vi "Lab Panel V5.28.vi"() -> ()   [LabVIEW 2013] (continued)
                  tunnel: w2122 -> [_ w2132]
                  frame False {
                  }
                  frame True {
                    n1115 = local read "SET LAB01-1"() -> (w2134:T5)
                    n1116 = local read "TDMS LAB01-1"() -> (w2127:refnum<k34>)
                    n1117 = Unbundle(w2134) -> ("CYCLES"=w2125:dbl, "T-RISE mins"=w2131:dbl)  [unwired: 3 out]
                    n1118 = case shown="\"CYCLE TEST\"" w2132 {
                      tunnel: w2131 -> [_ _ w2141]
                      tunnel: [w2136 w2138 w2141] -> w2130
                      tunnel: w2125 -> [w2136 w2138 _]
                      tunnel: ["CHART PASS" "CYCLE PASS" "T-RISE PASS"] -> w2129
                      frame "CHART TEST", Default {
                      }
                      frame "CYCLE TEST" {
                      }
                      frame "T-RISE TEST" {
                      }
                    }
                    n1119 = Unbundle(w2128) -> ("CYCLE"=w2133:dbl)  [unwired: 2 out]
                    n1120 = Increment(x=w2125) -> (x+1=w2126:dbl)
                    n1121 = Greater Or Equal?(x=w2133, y=w2126) -> (x >= y?=w2135:bool)
                    n1122 = case shown="True" w2135 {
                      tunnel: w2130 -> [w2145 _]
                      tunnel: w2129 -> [w2144 _]
                      tunnel: w2128 -> [w2143 _]
                      tunnel: w2127 -> [w2142 _]
                      frame True {
                        n1123 = stacked-sequence {
                          tunnel: w2145 -> [w2149 _]
                          tunnel: w2144 -> [w2147 w2153]
                          tunnel: w2143 -> [_ w2156]
                          tunnel: w2142 -> [w2146 _]
                          frame #0 {
                            n1124 = Build Array(w2147) -> (w2150:string[])
                            n1125 = Build Array(w2149) -> (w2148:dbl[])
                            n1126 = TDMS Write(0:w2146, 5:"TEST PASS", 7:w2150, 9:w2148) -> (15:w2152:errorcluster)  [unwired: 2 in, 3 out]
                            n1127 = local write "data file error"(w2152) -> ()
                          }
                          frame #1 {
                            n1128 = Bundle(cluster=w2156, "STATUS"=w2153) -> (w2154:T4)  [unwired: 2 in]
                            n1129 = local write "RESULT LAB01-1"(TRUE) -> ()
                            n1130 = local write "DISP LAB01-1"(w2154) -> ()
                          }
                        }
                      }
                      frame False {
                      }
                    }
                  }
                }
              }
              frame #1 {
                # "LAB01-2"
                n1131 = Less?(x=w2157, y=2) -> (x < y?=w2160:bool)
                n1132 = local read "DISP LAB01-2"() -> (w2162:T4)
                n1133 = Unbundle(w2162) -> ("STATUS"=w2163:string)  [unwired: 2 out]
                n1134 = Equal?(x=w2163, y="RUN") -> (x = y?=w2159:bool)
                n1135 = And(x=w2159, y=w2160) -> (x .and. y?=w2158:bool)
                n1136 = case shown="True" w2158 {
                  tunnel: w2162 -> [_ w2168]
                  tunnel: w2157 -> [_ w2172]
                  frame False {
                  }
                  frame True {
                    n1137 = local read "SET LAB01-2"() -> (w2174:T5)
                    n1138 = local read "TDMS LAB01-2"() -> (w2167:refnum<k34>)
                    n1139 = Unbundle(w2174) -> ("CYCLES"=w2165:dbl, "T-RISE mins"=w2171:dbl)  [unwired: 3 out]
                    n1140 = case shown="\"T-RISE TEST\"" w2172 {
                      tunnel: w2171 -> [_ _ w2181]
                      tunnel: [w2176 w2178 w2181] -> w2170
                      tunnel: w2165 -> [w2176 w2178 _]
                      tunnel: ["CHART PASS" "CYCLE PASS" "T-RISE PASS"] -> w2169
                      frame "CHART TEST", Default {
                      }
                      frame "CYCLE TEST" {
                      }
                      frame "T-RISE TEST" {
                      }
                    }
                    n1141 = Unbundle(w2168) -> ("CYCLE"=w2173:dbl)  [unwired: 2 out]
                    n1142 = Increment(x=w2165) -> (x+1=w2166:dbl)
                    n1143 = Greater Or Equal?(x=w2173, y=w2166) -> (x >= y?=w2175:bool)
                    n1144 = case shown="True" w2175 {
                      tunnel: w2170 -> [w2185 _]
                      tunnel: w2169 -> [w2184 _]
                      tunnel: w2168 -> [w2183 _]
                      tunnel: w2167 -> [w2182 _]
                      frame True {
                        n1145 = stacked-sequence {
                          tunnel: w2185 -> [w2189 _]
                          tunnel: w2184 -> [w2187 w2193]
                          tunnel: w2183 -> [_ w2196]
                          tunnel: w2182 -> [w2186 _]
                          frame #0 {
                            n1146 = Build Array(w2187) -> (w2190:string[])
                            n1147 = Build Array(w2189) -> (w2188:dbl[])
                            n1148 = TDMS Write(0:w2186, 5:"TEST PASS", 7:w2190, 9:w2188) -> (15:w2192:errorcluster)  [unwired: 2 in, 3 out]
                            n1149 = local write "data file error"(w2192) -> ()
                          }
                          frame #1 {
                            n1150 = Bundle(cluster=w2196, "STATUS"=w2193) -> (w2194:T4)  [unwired: 2 in]
                            n1151 = local write "RESULT LAB01-2"(TRUE) -> ()
                            n1152 = local write "DISP LAB01-2"(w2194) -> ()
                          }
                        }
                      }
                      frame False {
                      }
                    }
                  }
                }
              }
              frame #2 {
                # "LAB02-1"
                n1153 = Less?(x=w2197, y=2) -> (x < y?=w2200:bool)
                n1154 = local read "DISP LAB02-1"() -> (w2202:T4)
                n1155 = Unbundle(w2202) -> ("STATUS"=w2203:string)  [unwired: 2 out]
                n1156 = Equal?(x=w2203, y="RUN") -> (x = y?=w2199:bool)
                n1157 = And(x=w2199, y=w2200) -> (x .and. y?=w2198:bool)
                n1158 = case shown="True" w2198 {
                  tunnel: w2202 -> [_ w2208]
                  tunnel: w2197 -> [_ w2212]
                  frame False {
                  }
                  frame True {
                    n1159 = local read "SET LAB02-1"() -> (w2214:T5)
                    n1160 = local read "TDMS LAB02-1"() -> (w2207:refnum<k34>)
                    n1161 = Unbundle(w2208) -> ("CYCLE"=w2213:dbl)  [unwired: 2 out]
                    n1162 = Unbundle(w2214) -> ("CYCLES"=w2205:dbl, "T-RISE mins"=w2211:dbl)  [unwired: 3 out]
                    n1163 = case shown="\"T-RISE TEST\"" w2212 {
                      tunnel: w2211 -> [_ _ w2221]
                      tunnel: [w2216 w2218 w2221] -> w2210
                      tunnel: w2205 -> [w2216 w2218 _]
                      tunnel: ["CHART PASS" "CYCLE PASS" "T-RISE PASS"] -> w2209
                      frame "CHART TEST", Default {
                      }
                      frame "CYCLE TEST" {
                      }
                      frame "T-RISE TEST" {
                      }
                    }
                    n1164 = Increment(x=w2205) -> (x+1=w2206:dbl)
                    n1165 = Greater Or Equal?(x=w2213, y=w2206) -> (x >= y?=w2215:bool)
                    n1166 = case shown="True" w2215 {
                      tunnel: w2210 -> [w2225 _]
                      tunnel: w2209 -> [w2224 _]
                      tunnel: w2208 -> [w2223 _]
                      tunnel: w2207 -> [w2222 _]
                      frame True {
                        n1167 = stacked-sequence {
                          tunnel: w2225 -> [w2229 _]
                          tunnel: w2224 -> [w2227 w2233]
                          tunnel: w2223 -> [_ w2236]
                          tunnel: w2222 -> [w2226 _]
                          frame #0 {
                            n1168 = Build Array(w2227) -> (w2230:string[])
                            n1169 = Build Array(w2229) -> (w2228:dbl[])
                            n1170 = TDMS Write(0:w2226, 5:"TEST PASS", 7:w2230, 9:w2228) -> (15:w2232:errorcluster)  [unwired: 2 in, 3 out]
                            n1171 = local write "data file error"(w2232) -> ()
                          }
                          frame #1 {
                            n1172 = Bundle(cluster=w2236, "STATUS"=w2233) -> (w2234:T4)  [unwired: 2 in]
                            n1173 = local write "RESULT LAB02-1"(TRUE) -> ()
                            n1174 = local write "DISP LAB02-1"(w2234) -> ()
                          }
                        }
                      }
                      frame False {
                      }
                    }
                  }
                }
              }
              frame #3 {
                # "LAB02-2"
                n1175 = Less?(x=w2237, y=2) -> (x < y?=w2240:bool)
                n1176 = local read "DISP LAB02-2"() -> (w2242:T4)
                n1177 = Unbundle(w2242) -> ("STATUS"=w2243:string)  [unwired: 2 out]
                n1178 = Equal?(x=w2243, y="RUN") -> (x = y?=w2239:bool)
                n1179 = And(x=w2239, y=w2240) -> (x .and. y?=w2238:bool)
                n1180 = case shown="True" w2238 {
                  tunnel: w2242 -> [_ w2248]
                  tunnel: w2237 -> [_ w2252]
                  frame False {
                  }
                  frame True {
                    n1181 = local read "SET LAB02-2"() -> (w2254:T5)
                    n1182 = local read "TDMS LAB02-2"() -> (w2247:refnum<k34>)
                    n1183 = Unbundle(w2248) -> ("CYCLE"=w2253:dbl)  [unwired: 2 out]
                    n1184 = Unbundle(w2254) -> ("CYCLES"=w2245:dbl, "T-RISE mins"=w2251:dbl)  [unwired: 3 out]
                    n1185 = case shown="\"T-RISE TEST\"" w2252 {
                      tunnel: w2251 -> [_ _ w2261]
                      tunnel: [w2256 w2258 w2261] -> w2250
                      tunnel: w2245 -> [w2256 w2258 _]
                      tunnel: ["CHART PASS" "CYCLE PASS" "T-RISE PASS"] -> w2249
                      frame "CHART TEST", Default {
                      }
                      frame "CYCLE TEST" {
                      }
                      frame "T-RISE TEST" {
                      }
                    }
                    n1186 = Increment(x=w2245) -> (x+1=w2246:dbl)
                    n1187 = Greater Or Equal?(x=w2253, y=w2246) -> (x >= y?=w2255:bool)
                    n1188 = case shown="True" w2255 {
                      tunnel: w2250 -> [w2265 _]
                      tunnel: w2249 -> [w2264 _]
                      tunnel: w2248 -> [w2263 _]
                      tunnel: w2247 -> [w2262 _]
                      frame True {
                        n1189 = stacked-sequence {
                          tunnel: w2265 -> [w2269 _]
                          tunnel: w2264 -> [w2267 w2273]
                          tunnel: w2263 -> [_ w2276]
                          tunnel: w2262 -> [w2266 _]
                          frame #0 {
                            n1190 = Build Array(w2267) -> (w2270:string[])
                            n1191 = Build Array(w2269) -> (w2268:dbl[])
                            n1192 = TDMS Write(0:w2266, 5:"TEST PASS", 7:w2270, 9:w2268) -> (15:w2272:errorcluster)  [unwired: 2 in, 3 out]
                            n1193 = local write "data file error"(w2272) -> ()
                          }
                          frame #1 {
                            n1194 = Bundle(cluster=w2276, "STATUS"=w2273) -> (w2274:T4)  [unwired: 2 in]
                            n1195 = local write "RESULT LAB02-2"(TRUE) -> ()
                            n1196 = local write "DISP LAB02-2"(w2274) -> ()
                          }
                        }
                      }
                      frame False {
                      }
                    }
                  }
                }
              }
              frame #4 {
                # "LAB03-1"
                n1197 = Less?(x=w2277, y=2) -> (x < y?=w2280:bool)
                n1198 = local read "DISP LAB03-1"() -> (w2282:T4)
                n1199 = Unbundle(w2282) -> ("STATUS"=w2283:string)  [unwired: 2 out]
                n1200 = Equal?(x=w2283, y="RUN") -> (x = y?=w2279:bool)
                n1201 = And(x=w2279, y=w2280) -> (x .and. y?=w2278:bool)
                n1202 = case shown="True" w2278 {
                  tunnel: w2282 -> [_ w2288]
                  tunnel: w2277 -> [_ w2292]
                  frame False {
                  }
                  frame True {
                    n1203 = local read "SET LAB03-1"() -> (w2294:T5)
                    n1204 = local read "TDMS LAB03-1"() -> (w2287:refnum<k34>)
                    n1205 = Unbundle(w2288) -> ("CYCLE"=w2293:dbl)  [unwired: 2 out]
                    n1206 = Unbundle(w2294) -> ("CYCLES"=w2285:dbl, "T-RISE mins"=w2291:dbl)  [unwired: 3 out]
                    n1207 = case shown="\"T-RISE TEST\"" w2292 {
                      tunnel: w2291 -> [_ _ w2301]
                      tunnel: [w2296 w2298 w2301] -> w2290
                      tunnel: w2285 -> [w2296 w2298 _]
                      tunnel: ["CHART PASS" "CYCLE PASS" "T-RISE PASS"] -> w2289
                      frame "CHART TEST", Default {
                      }
                      frame "CYCLE TEST" {
                      }
                      frame "T-RISE TEST" {
                      }
                    }
                    n1208 = Increment(x=w2285) -> (x+1=w2286:dbl)
                    n1209 = Greater Or Equal?(x=w2293, y=w2286) -> (x >= y?=w2295:bool)
                    n1210 = case shown="True" w2295 {
                      tunnel: w2290 -> [w2305 _]
                      tunnel: w2289 -> [w2304 _]
                      tunnel: w2288 -> [w2303 _]
                      tunnel: w2287 -> [w2302 _]
                      frame True {
                        n1211 = stacked-sequence {
                          tunnel: w2305 -> [w2309 _]
                          tunnel: w2304 -> [w2307 w2313]
                          tunnel: w2303 -> [_ w2316]
                          tunnel: w2302 -> [w2306 _]
                          frame #0 {
                            n1212 = Build Array(w2307) -> (w2310:string[])
                            n1213 = Build Array(w2309) -> (w2308:dbl[])
                            n1214 = TDMS Write(0:w2306, 5:"TEST PASS", 7:w2310, 9:w2308) -> (15:w2312:errorcluster)  [unwired: 2 in, 3 out]
                            n1215 = local write "data file error"(w2312) -> ()
                          }
                          frame #1 {
                            n1216 = Bundle(cluster=w2316, "STATUS"=w2313) -> (w2314:T4)  [unwired: 2 in]
                            n1217 = local write "RESULT LAB03-1"(TRUE) -> ()
                            n1218 = local write "DISP LAB03-1"(w2314) -> ()
                          }
                        }
                      }
                      frame False {
                      }
                    }
                  }
                }
              }
              frame #5 {
                # "LAB03-2"
                n1219 = Less?(x=w2317, y=2) -> (x < y?=w2320:bool)
                n1220 = local read "DISP LAB03-2"() -> (w2322:T4)
                n1221 = Unbundle(w2322) -> ("STATUS"=w2323:string)  [unwired: 2 out]
                n1222 = Equal?(x=w2323, y="RUN") -> (x = y?=w2319:bool)
                n1223 = And(x=w2319, y=w2320) -> (x .and. y?=w2318:bool)
                n1224 = case shown="True" w2318 {
                  tunnel: w2322 -> [_ w2328]
                  tunnel: w2317 -> [_ w2332]
                  frame False {
                  }
                  frame True {
                    n1225 = local read "SET LAB03-2"() -> (w2334:T5)
                    n1226 = local read "TDMS LAB03-2"() -> (w2327:refnum<k34>)
                    n1227 = Unbundle(w2328) -> ("CYCLE"=w2333:dbl)  [unwired: 2 out]
                    n1228 = Unbundle(w2334) -> ("CYCLES"=w2325:dbl, "T-RISE mins"=w2331:dbl)  [unwired: 3 out]
                    n1229 = case shown="\"T-RISE TEST\"" w2332 {
                      tunnel: w2331 -> [_ _ w2341]
                      tunnel: [w2336 w2338 w2341] -> w2330
                      tunnel: w2325 -> [w2336 w2338 _]
                      tunnel: ["CHART PASS" "CYCLE PASS" "T-RISE PASS"] -> w2329
                      frame "CHART TEST", Default {
                      }
                      frame "CYCLE TEST" {
                      }
                      frame "T-RISE TEST" {
                      }
                    }
                    n1230 = Increment(x=w2325) -> (x+1=w2326:dbl)
                    n1231 = Greater Or Equal?(x=w2333, y=w2326) -> (x >= y?=w2335:bool)
                    n1232 = case shown="True" w2335 {
                      tunnel: w2330 -> [w2345 _]
                      tunnel: w2329 -> [w2344 _]
                      tunnel: w2328 -> [w2343 _]
                      tunnel: w2327 -> [w2342 _]
                      frame True {
                        n1233 = stacked-sequence {
                          tunnel: w2345 -> [w2349 _]
                          tunnel: w2344 -> [w2347 w2353]
                          tunnel: w2343 -> [_ w2356]
                          tunnel: w2342 -> [w2346 _]
                          frame #0 {
                            n1234 = Build Array(w2347) -> (w2350:string[])
                            n1235 = Build Array(w2349) -> (w2348:dbl[])
                            n1236 = TDMS Write(0:w2346, 5:"TEST PASS", 7:w2350, 9:w2348) -> (15:w2352:errorcluster)  [unwired: 2 in, 3 out]
                            n1237 = local write "data file error"(w2352) -> ()
                          }
                          frame #1 {
                            n1238 = Bundle(cluster=w2356, "STATUS"=w2353) -> (w2354:T4)  [unwired: 2 in]
                            n1239 = local write "RESULT LAB03-2"(TRUE) -> ()
                            n1240 = local write "DISP LAB03-2"(w2354) -> ()
                          }
                        }
                      }
                      frame False {
                      }
                    }
                  }
                }
              }
              frame #6 {
                # "LAB04-1"
                n1241 = Less?(x=w2357, y=2) -> (x < y?=w2360:bool)
                n1242 = local read "DISP LAB04-1"() -> (w2362:T4)
                n1243 = Unbundle(w2362) -> ("STATUS"=w2363:string)  [unwired: 2 out]
                n1244 = Equal?(x=w2363, y="RUN") -> (x = y?=w2359:bool)
                n1245 = And(x=w2359, y=w2360) -> (x .and. y?=w2358:bool)
                n1246 = case shown="True" w2358 {
                  tunnel: w2362 -> [_ w2368]
                  tunnel: w2357 -> [_ w2372]
                  frame False {
                  }
                  frame True {
                    n1247 = local read "SET LAB04-1"() -> (w2374:T5)
                    n1248 = local read "TDMS LAB04-1"() -> (w2367:refnum<k34>)
                    n1249 = Unbundle(w2368) -> ("CYCLE"=w2373:dbl)  [unwired: 2 out]
                    n1250 = Unbundle(w2374) -> ("CYCLES"=w2365:dbl, "T-RISE mins"=w2371:dbl)  [unwired: 3 out]
                    n1251 = case shown="\"T-RISE TEST\"" w2372 {
                      tunnel: w2371 -> [_ _ w2381]
                      tunnel: [w2376 w2378 w2381] -> w2370
                      tunnel: w2365 -> [w2376 w2378 _]
                      tunnel: ["CHART PASS" "CYCLE PASS" "T-RISE PASS"] -> w2369
                      frame "CHART TEST", Default {
                      }
                      frame "CYCLE TEST" {
                      }
                      frame "T-RISE TEST" {
                      }
                    }
                    n1252 = Increment(x=w2365) -> (x+1=w2366:dbl)
                    n1253 = Greater Or Equal?(x=w2373, y=w2366) -> (x >= y?=w2375:bool)
                    n1254 = case shown="True" w2375 {
                      tunnel: w2370 -> [w2385 _]
                      tunnel: w2369 -> [w2384 _]
                      tunnel: w2368 -> [w2383 _]
                      tunnel: w2367 -> [w2382 _]
                      frame True {
                        n1255 = stacked-sequence {
                          tunnel: w2385 -> [w2389 _]
                          tunnel: w2384 -> [w2387 w2393]
                          tunnel: w2383 -> [_ w2396]
                          tunnel: w2382 -> [w2386 _]
                          frame #0 {
                            n1256 = Build Array(w2387) -> (w2390:string[])
                            n1257 = Build Array(w2389) -> (w2388:dbl[])
                            n1258 = TDMS Write(0:w2386, 5:"TEST PASS", 7:w2390, 9:w2388) -> (15:w2392:errorcluster)  [unwired: 2 in, 3 out]
                            n1259 = local write "data file error"(w2392) -> ()
                          }
                          frame #1 {
                            n1260 = Bundle(cluster=w2396, "STATUS"=w2393) -> (w2394:T4)  [unwired: 2 in]
                            n1261 = local write "RESULT LAB04-1"(TRUE) -> ()
                            n1262 = local write "DISP LAB04-1"(w2394) -> ()
                          }
                        }
                      }
                      frame False {
                      }
                    }
                  }
                }
              }
              frame #7 {
                # "LAB04-2"
                n1263 = Less?(x=w2397, y=2) -> (x < y?=w2400:bool)
                n1264 = local read "DISP LAB04-2"() -> (w2402:T4)
                n1265 = Unbundle(w2402) -> ("STATUS"=w2403:string)  [unwired: 2 out]
                n1266 = Equal?(x=w2403, y="RUN") -> (x = y?=w2399:bool)
                n1267 = And(x=w2399, y=w2400) -> (x .and. y?=w2398:bool)
                n1268 = case shown="True" w2398 {
                  tunnel: w2402 -> [_ w2408]
                  tunnel: w2397 -> [_ w2412]
                  frame False {
                  }
                  frame True {
                    n1269 = local read "SET LAB04-2"() -> (w2414:T5)
                    n1270 = local read "TDMS LAB04-2"() -> (w2407:refnum<k34>)
                    n1271 = Unbundle(w2408) -> ("CYCLE"=w2413:dbl)  [unwired: 2 out]
                    n1272 = Unbundle(w2414) -> ("CYCLES"=w2405:dbl, "T-RISE mins"=w2411:dbl)  [unwired: 3 out]
                    n1273 = case shown="\"T-RISE TEST\"" w2412 {
                      tunnel: w2411 -> [_ _ w2421]
                      tunnel: [w2416 w2418 w2421] -> w2410
                      tunnel: w2405 -> [w2416 w2418 _]
                      tunnel: ["CHART PASS" "CYCLE PASS" "T-RISE PASS"] -> w2409
                      frame "CHART TEST", Default {
                      }
                      frame "CYCLE TEST" {
                      }
                      frame "T-RISE TEST" {
                      }
                    }
                    n1274 = Increment(x=w2405) -> (x+1=w2406:dbl)
                    n1275 = Greater Or Equal?(x=w2413, y=w2406) -> (x >= y?=w2415:bool)
                    n1276 = case shown="True" w2415 {
                      tunnel: w2410 -> [w2425 _]
                      tunnel: w2409 -> [w2424 _]
                      tunnel: w2408 -> [w2423 _]
                      tunnel: w2407 -> [w2422 _]
                      frame True {
                        n1277 = stacked-sequence {
                          tunnel: w2425 -> [w2429 _]
                          tunnel: w2424 -> [w2427 w2433]
                          tunnel: w2423 -> [_ w2436]
                          tunnel: w2422 -> [w2426 _]
                          frame #0 {
                            n1278 = Build Array(w2427) -> (w2430:string[])
                            n1279 = Build Array(w2429) -> (w2428:dbl[])
                            n1280 = TDMS Write(0:w2426, 5:"TEST PASS", 7:w2430, 9:w2428) -> (15:w2432:errorcluster)  [unwired: 2 in, 3 out]
                            n1281 = local write "data file error"(w2432) -> ()
                          }
                          frame #1 {
                            n1282 = Bundle(cluster=w2436, "STATUS"=w2433) -> (w2434:T4)  [unwired: 2 in]
                            n1283 = local write "RESULT LAB04-2"(TRUE) -> ()
                            n1284 = local write "DISP LAB04-2"(w2434) -> ()
                          }
                        }
                      }
                      frame False {
                      }
                    }
                  }
                }
              }
              frame #8 {
                # "LAB05-1"
                n1285 = Less?(x=w2437, y=2) -> (x < y?=w2440:bool)
                n1286 = local read "DISP LAB05-1"() -> (w2442:T4)
                n1287 = Unbundle(w2442) -> ("STATUS"=w2443:string)  [unwired: 2 out]
                n1288 = Equal?(x=w2443, y="RUN") -> (x = y?=w2439:bool)
                n1289 = And(x=w2439, y=w2440) -> (x .and. y?=w2438:bool)
                n1290 = case shown="True" w2438 {
                  tunnel: w2442 -> [_ w2448]
                  tunnel: w2437 -> [_ w2452]
                  frame False {
                  }
                  frame True {
                    n1291 = local read "SET LAB05-1"() -> (w2454:T5)
                    n1292 = local read "TDMS LAB05-1"() -> (w2447:refnum<k34>)
                    n1293 = Unbundle(w2448) -> ("CYCLE"=w2453:dbl)  [unwired: 2 out]
                    n1294 = Unbundle(w2454) -> ("CYCLES"=w2445:dbl, "T-RISE mins"=w2451:dbl)  [unwired: 3 out]
                    n1295 = case shown="\"T-RISE TEST\"" w2452 {
                      tunnel: w2451 -> [_ _ w2461]
                      tunnel: [w2456 w2458 w2461] -> w2450
                      tunnel: w2445 -> [w2456 w2458 _]
                      tunnel: ["CHART PASS" "CYCLE PASS" "T-RISE PASS"] -> w2449
                      frame "CHART TEST", Default {
                      }
                      frame "CYCLE TEST" {
                      }
                      frame "T-RISE TEST" {
                      }
                    }
                    n1296 = Increment(x=w2445) -> (x+1=w2446:dbl)
                    n1297 = Greater Or Equal?(x=w2453, y=w2446) -> (x >= y?=w2455:bool)
                    n1298 = case shown="True" w2455 {
                      tunnel: w2450 -> [w2465 _]
                      tunnel: w2449 -> [w2464 _]
                      tunnel: w2448 -> [w2463 _]
                      tunnel: w2447 -> [w2462 _]
                      frame True {
                        n1299 = stacked-sequence {
                          tunnel: w2465 -> [w2469 _]
                          tunnel: w2464 -> [w2467 w2473]
                          tunnel: w2463 -> [_ w2476]
                          tunnel: w2462 -> [w2466 _]
                          frame #0 {
                            n1300 = Build Array(w2467) -> (w2470:string[])
                            n1301 = Build Array(w2469) -> (w2468:dbl[])
                            n1302 = TDMS Write(0:w2466, 5:"TEST PASS", 7:w2470, 9:w2468) -> (15:w2472:errorcluster)  [unwired: 2 in, 3 out]
                            n1303 = local write "data file error"(w2472) -> ()
                          }
                          frame #1 {
                            n1304 = Bundle(cluster=w2476, "STATUS"=w2473) -> (w2474:T4)  [unwired: 2 in]
                            n1305 = local write "RESULT LAB05-1"(TRUE) -> ()
                            n1306 = local write "DISP LAB05-1"(w2474) -> ()
                          }
                        }
                      }
                      frame False {
                      }
                    }
                  }
                }
              }
              frame #9 {
                # "LAB05-2"
                n1307 = Less?(x=w2477, y=2) -> (x < y?=w2480:bool)
                n1308 = local read "DISP LAB05-2"() -> (w2482:T4)
                n1309 = Unbundle(w2482) -> ("STATUS"=w2483:string)  [unwired: 2 out]
                n1310 = Equal?(x=w2483, y="RUN") -> (x = y?=w2479:bool)
                n1311 = And(x=w2479, y=w2480) -> (x .and. y?=w2478:bool)
                n1312 = case shown="True" w2478 {
                  tunnel: w2482 -> [_ w2488]
                  tunnel: w2477 -> [_ w2492]
                  frame False {
                  }
                  frame True {
                    n1313 = local read "SET LAB05-2"() -> (w2494:T5)
                    n1314 = local read "TDMS LAB05-2"() -> (w2487:refnum<k34>)
                    n1315 = Unbundle(w2488) -> ("CYCLE"=w2493:dbl)  [unwired: 2 out]
                    n1316 = Unbundle(w2494) -> ("CYCLES"=w2485:dbl, "T-RISE mins"=w2491:dbl)  [unwired: 3 out]
                    n1317 = case shown="\"T-RISE TEST\"" w2492 {
                      tunnel: w2491 -> [_ _ w2501]
                      tunnel: [w2496 w2498 w2501] -> w2490
                      tunnel: w2485 -> [w2496 w2498 _]
                      tunnel: ["CHART PASS" "CYCLE PASS" "T-RISE PASS"] -> w2489
                      frame "CHART TEST", Default {
                      }
                      frame "CYCLE TEST" {
                      }
                      frame "T-RISE TEST" {
                      }
                    }
                    n1318 = Increment(x=w2485) -> (x+1=w2486:dbl)
                    n1319 = Greater Or Equal?(x=w2493, y=w2486) -> (x >= y?=w2495:bool)
                    n1320 = case shown="True" w2495 {
                      tunnel: w2490 -> [w2505 _]
                      tunnel: w2489 -> [w2504 _]
                      tunnel: w2488 -> [w2503 _]
                      tunnel: w2487 -> [w2502 _]
                      frame True {
                        n1321 = stacked-sequence {
                          tunnel: w2505 -> [w2509 _]
                          tunnel: w2504 -> [w2507 w2513]
                          tunnel: w2503 -> [_ w2516]
                          tunnel: w2502 -> [w2506 _]
                          frame #0 {
                            n1322 = Build Array(w2507) -> (w2510:string[])
                            n1323 = Build Array(w2509) -> (w2508:dbl[])
                            n1324 = TDMS Write(0:w2506, 5:"TEST PASS", 7:w2510, 9:w2508) -> (15:w2512:errorcluster)  [unwired: 2 in, 3 out]
                            n1325 = local write "data file error"(w2512) -> ()
                          }
                          frame #1 {
                            n1326 = Bundle(cluster=w2516, "STATUS"=w2513) -> (w2514:T4)  [unwired: 2 in]
                            n1327 = local write "RESULT LAB05-2"(TRUE) -> ()
                            n1328 = local write "DISP LAB05-2"(w2514) -> ()
                          }
                        }
                      }
                      frame False {
                      }
                    }
                  }
                }
              }
            }
          }
          frame #6 {
            # "check if test cycles reached for temperature rise test"
            n1329 = stacked-sequence {
              tunnel: w2546 -> [_ _ _ _ _ _ _ _ _ _]
              tunnel: w2545 -> [_ _ _ _ _ _ _ _ _ _]
              tunnel: w2544 -> [_ _ _ _ _ _ _ _ _ _]
              tunnel: w2543 -> [_ _ _ _ _ _ _ _ _ _]
              tunnel: w2542 -> [_ _ _ _ _ _ _ _ _ _]
              tunnel: w2541 -> [_ _ _ _ _ _ _ _ _ _]
              tunnel: w2540 -> [_ _ _ _ _ _ _ _ _ _]
              tunnel: w2539 -> [_ _ _ _ _ _ _ _ _ _]
              tunnel: w2538 -> [_ _ _ _ _ _ _ _ _ _]
              tunnel: w2537 -> [_ _ _ _ _ _ _ _ _ _]
              tunnel: w2536 -> [w2552 _ _ _ _ _ _ _ _ _]
              tunnel: w2526 -> [w2547 _ _ _ _ _ _ _ _ _]
              tunnel: w2535 -> [_ w2578 _ _ _ _ _ _ _ _]
              tunnel: w2534 -> [_ _ w2608 _ _ _ _ _ _ _]
              tunnel: w2533 -> [_ _ _ w2638 _ _ _ _ _ _]
              tunnel: w2532 -> [_ _ _ _ w2668 _ _ _ _ _]
              tunnel: w2531 -> [_ _ _ _ _ w2698 _ _ _ _]
              tunnel: w2530 -> [_ _ _ _ _ _ w2728 _ _ _]
              tunnel: w2529 -> [_ _ _ _ _ _ _ w2758 _ _]
              tunnel: w2528 -> [_ _ _ _ _ _ _ _ w2788 _]
              tunnel: w2527 -> [_ _ _ _ _ _ _ _ _ w2818]
              tunnel: w2525 -> [_ w2577 _ _ _ _ _ _ _ _]
              tunnel: w2524 -> [_ _ w2607 _ _ _ _ _ _ _]
              tunnel: w2523 -> [_ _ _ w2637 _ _ _ _ _ _]
              tunnel: w2522 -> [_ _ _ _ w2667 _ _ _ _ _]
              tunnel: w2521 -> [_ _ _ _ _ w2697 _ _ _ _]
              tunnel: w2520 -> [_ _ _ _ _ _ w2727 _ _ _]
              tunnel: w2519 -> [_ _ _ _ _ _ _ w2757 _ _]
              tunnel: w2518 -> [_ _ _ _ _ _ _ _ w2787 _]
              tunnel: w2517 -> [_ _ _ _ _ _ _ _ _ w2817]
              frame #0 {
                # "LAB01-1"
                n1330 = Equal?(x=w2552, y=2) -> (x = y?=w2550:bool)
                n1331 = local read "DISP LAB01-1"() -> (w2553:T4)
                n1332 = Unbundle(w2553) -> ("STATUS"=w2554:string)  [unwired: 2 out]
                n1333 = Equal?(x=w2554, y="RUN") -> (x = y?=w2549:bool)
                n1334 = And(x=w2549, y=w2550) -> (x .and. y?=w2548:bool)
                n1335 = case shown="True" w2548 {
                  tunnel: w2553 -> [_ w2557]
                  tunnel: w2547 -> [_ w2560]
                  frame False {
                  }
                  frame True {
                    n1336 = local read "SET LAB01-1"() -> (w2559:T5)
                    n1337 = local read "TDMS LAB01-1"() -> (w2556:refnum<k34>)
                    n1338 = Unbundle(w2557) -> ("CYCLE"=w2561:dbl)  [unwired: 2 out]
                    n1339 = Unbundle(w2559) -> ("T-RISE mins"=w2558:dbl)  [unwired: 4 out]
                    n1340 = Greater Or Equal?(x=w2561, y=w2560) -> (x >= y?=w2562:bool)
                    n1341 = case shown="True" w2562 {
                      tunnel: w2558 -> [w2565 _]
                      tunnel: w2557 -> [w2564 _]
                      tunnel: w2556 -> [w2563 _]
                      frame True {
                        n1342 = stacked-sequence {
                          tunnel: w2565 -> [w2568 _]
                          tunnel: w2564 -> [_ w2573]
                          tunnel: w2563 -> [w2566 _]
                          frame #0 {
                            n1343 = Build Array("T-RISE") -> (w2570:string[])
                            n1344 = Build Array(w2568) -> (w2569:dbl[])
                            n1345 = TDMS Write(0:w2566, 5:"TEST PASS", 7:w2570, 9:w2569) -> (15:w2572:errorcluster)  [unwired: 2 in, 3 out]
                            n1346 = local write "data file error"(w2572) -> ()
                          }
                          frame #1 {
                            n1347 = Bundle(cluster=w2573, "STATUS"="T-RISE PASS") -> (w2575:T4)  [unwired: 2 in]
                            n1348 = local write "RESULT LAB01-1"(TRUE) -> ()
                            n1349 = local write "DISP LAB01-1"(w2575) -> ()
                          }
                        }
                      }
                      frame False {
                      }
                    }
                  }
                }
              }
              frame #1 {
                # "LAB01-2"
                n1350 = Equal?(x=w2578, y=2) -> (x = y?=w2581:bool)
                n1351 = local read "DISP LAB01-2"() -> (w2583:T4)
                n1352 = Unbundle(w2583) -> ("STATUS"=w2584:string)  [unwired: 2 out]
                n1353 = Equal?(x=w2584, y="RUN") -> (x = y?=w2580:bool)
                n1354 = And(x=w2580, y=w2581) -> (x .and. y?=w2579:bool)
                n1355 = case shown="True" w2579 {
                  tunnel: w2583 -> [_ w2587]
                  tunnel: w2577 -> [_ w2590]
                  frame False {
                  }
                  frame True {
                    n1356 = local read "SET LAB01-2"() -> (w2589:T5)
                    n1357 = local read "TDMS LAB01-2"() -> (w2586:refnum<k34>)
                    n1358 = Unbundle(w2587) -> ("CYCLE"=w2591:dbl)  [unwired: 2 out]
                    n1359 = Unbundle(w2589) -> ("T-RISE mins"=w2588:dbl)  [unwired: 4 out]
                    n1360 = Greater Or Equal?(x=w2591, y=w2590) -> (x >= y?=w2592:bool)
                    n1361 = case shown="True" w2592 {
                      tunnel: w2588 -> [w2595 _]
                      tunnel: w2587 -> [w2594 _]
                      tunnel: w2586 -> [w2593 _]
                      frame True {
                        n1362 = stacked-sequence {
                          tunnel: w2595 -> [w2598 _]
                          tunnel: w2594 -> [_ w2603]
                          tunnel: w2593 -> [w2596 _]
                          frame #0 {
                            n1363 = Build Array("T-RISE") -> (w2600:string[])
                            n1364 = Build Array(w2598) -> (w2599:dbl[])
                            n1365 = TDMS Write(0:w2596, 5:"TEST PASS", 7:w2600, 9:w2599) -> (15:w2602:errorcluster)  [unwired: 2 in, 3 out]
                            n1366 = local write "data file error"(w2602) -> ()
                          }
                          frame #1 {
                            n1367 = Bundle(cluster=w2603, "STATUS"="T-RISE PASS") -> (w2605:T4)  [unwired: 2 in]
                            n1368 = local write "RESULT LAB01-2"(TRUE) -> ()
                            n1369 = local write "DISP LAB01-2"(w2605) -> ()
                          }
                        }
                      }
                      frame False {
                      }
                    }
                  }
                }
              }
              frame #2 {
                # "LAB02-1"
                n1370 = Equal?(x=w2608, y=2) -> (x = y?=w2611:bool)
                n1371 = local read "DISP LAB02-1"() -> (w2613:T4)
                n1372 = Unbundle(w2613) -> ("STATUS"=w2614:string)  [unwired: 2 out]
                n1373 = Equal?(x=w2614, y="RUN") -> (x = y?=w2610:bool)
                n1374 = And(x=w2610, y=w2611) -> (x .and. y?=w2609:bool)
                n1375 = case shown="True" w2609 {
                  tunnel: w2613 -> [_ w2617]
                  tunnel: w2607 -> [_ w2620]
                  frame False {
                  }
                  frame True {
                    n1376 = local read "SET LAB02-1"() -> (w2619:T5)
                    n1377 = local read "TDMS LAB02-1"() -> (w2616:refnum<k34>)
                    n1378 = Unbundle(w2617) -> ("CYCLE"=w2621:dbl)  [unwired: 2 out]
                    n1379 = Unbundle(w2619) -> ("T-RISE mins"=w2618:dbl)  [unwired: 4 out]
                    n1380 = Greater Or Equal?(x=w2621, y=w2620) -> (x >= y?=w2622:bool)
                    n1381 = case shown="True" w2622 {
                      tunnel: w2618 -> [w2625 _]
                      tunnel: w2617 -> [w2624 _]
                      tunnel: w2616 -> [w2623 _]
                      frame True {
                        n1382 = stacked-sequence {
                          tunnel: w2625 -> [w2628 _]
                          tunnel: w2624 -> [_ w2633]
                          tunnel: w2623 -> [w2626 _]
                          frame #0 {
                            n1383 = Build Array("T-RISE") -> (w2630:string[])
                            n1384 = Build Array(w2628) -> (w2629:dbl[])
                            n1385 = TDMS Write(0:w2626, 5:"TEST PASS", 7:w2630, 9:w2629) -> (15:w2632:errorcluster)  [unwired: 2 in, 3 out]
                            n1386 = local write "data file error"(w2632) -> ()
                          }
                          frame #1 {
                            n1387 = Bundle(cluster=w2633, "STATUS"="T-RISE PASS") -> (w2635:T4)  [unwired: 2 in]
                            n1388 = local write "RESULT LAB02-1"(TRUE) -> ()
                            n1389 = local write "DISP LAB02-1"(w2635) -> ()
                          }
                        }
                      }
                      frame False {
                      }
                    }
                  }
                }
              }
              frame #3 {
                # "LAB02-2"
                n1390 = Equal?(x=w2638, y=2) -> (x = y?=w2641:bool)
                n1391 = local read "DISP LAB02-2"() -> (w2643:T4)
                n1392 = Unbundle(w2643) -> ("STATUS"=w2644:string)  [unwired: 2 out]
                n1393 = Equal?(x=w2644, y="RUN") -> (x = y?=w2640:bool)
                n1394 = And(x=w2640, y=w2641) -> (x .and. y?=w2639:bool)
                n1395 = case shown="True" w2639 {
                  tunnel: w2643 -> [_ w2647]
                  tunnel: w2637 -> [_ w2650]
                  frame False {
                  }
                  frame True {
                    n1396 = local read "SET LAB02-2"() -> (w2649:T5)
                    n1397 = local read "TDMS LAB02-2"() -> (w2646:refnum<k34>)
                    n1398 = Unbundle(w2647) -> ("CYCLE"=w2651:dbl)  [unwired: 2 out]
                    n1399 = Unbundle(w2649) -> ("T-RISE mins"=w2648:dbl)  [unwired: 4 out]
                    n1400 = Greater Or Equal?(x=w2651, y=w2650) -> (x >= y?=w2652:bool)
                    n1401 = case shown="True" w2652 {
                      tunnel: w2648 -> [w2655 _]
                      tunnel: w2647 -> [w2654 _]
                      tunnel: w2646 -> [w2653 _]
                      frame True {
                        n1402 = stacked-sequence {
                          tunnel: w2655 -> [w2658 _]
                          tunnel: w2654 -> [_ w2663]
                          tunnel: w2653 -> [w2656 _]
                          frame #0 {
                            n1403 = Build Array("T-RISE") -> (w2660:string[])
                            n1404 = Build Array(w2658) -> (w2659:dbl[])
                            n1405 = TDMS Write(0:w2656, 5:"TEST PASS", 7:w2660, 9:w2659) -> (15:w2662:errorcluster)  [unwired: 2 in, 3 out]
                            n1406 = local write "data file error"(w2662) -> ()
                          }
                          frame #1 {
                            n1407 = Bundle(cluster=w2663, "STATUS"="T-RISE PASS") -> (w2665:T4)  [unwired: 2 in]
                            n1408 = local write "RESULT LAB02-2"(TRUE) -> ()
                            n1409 = local write "DISP LAB02-2"(w2665) -> ()
                          }
                        }
                      }
                      frame False {
                      }
                    }
                  }
                }
              }
              frame #4 {
                # "LAB03-1"
                n1410 = Equal?(x=w2668, y=2) -> (x = y?=w2671:bool)
                n1411 = local read "DISP LAB03-1"() -> (w2673:T4)
                n1412 = Unbundle(w2673) -> ("STATUS"=w2674:string)  [unwired: 2 out]
                n1413 = Equal?(x=w2674, y="RUN") -> (x = y?=w2670:bool)
                n1414 = And(x=w2670, y=w2671) -> (x .and. y?=w2669:bool)
                n1415 = case shown="True" w2669 {
                  tunnel: w2673 -> [_ w2677]
                  tunnel: w2667 -> [_ w2680]
                  frame False {
                  }
                  frame True {
                    n1416 = local read "SET LAB03-1"() -> (w2679:T5)
                    n1417 = local read "TDMS LAB03-1"() -> (w2676:refnum<k34>)
                    n1418 = Unbundle(w2677) -> ("CYCLE"=w2681:dbl)  [unwired: 2 out]
                    n1419 = Unbundle(w2679) -> ("T-RISE mins"=w2678:dbl)  [unwired: 4 out]
                    n1420 = Greater Or Equal?(x=w2681, y=w2680) -> (x >= y?=w2682:bool)
                    n1421 = case shown="True" w2682 {
                      tunnel: w2678 -> [w2685 _]
                      tunnel: w2677 -> [w2684 _]
                      tunnel: w2676 -> [w2683 _]
                      frame True {
                        n1422 = stacked-sequence {
                          tunnel: w2685 -> [w2688 _]
                          tunnel: w2684 -> [_ w2693]
                          tunnel: w2683 -> [w2686 _]
                          frame #0 {
                            n1423 = Build Array("T-RISE") -> (w2690:string[])
                            n1424 = Build Array(w2688) -> (w2689:dbl[])
                            n1425 = TDMS Write(0:w2686, 5:"TEST PASS", 7:w2690, 9:w2689) -> (15:w2692:errorcluster)  [unwired: 2 in, 3 out]
                            n1426 = local write "data file error"(w2692) -> ()
                          }
                          frame #1 {
                            n1427 = Bundle(cluster=w2693, "STATUS"="T-RISE PASS") -> (w2695:T4)  [unwired: 2 in]
                            n1428 = local write "RESULT LAB03-1"(TRUE) -> ()
                            n1429 = local write "DISP LAB03-1"(w2695) -> ()
                          }
                        }
                      }
                      frame False {
                      }
                    }
                  }
                }
              }
              frame #5 {
                # "LAB03-2"
                n1430 = Equal?(x=w2698, y=2) -> (x = y?=w2701:bool)
                n1431 = local read "DISP LAB03-2"() -> (w2703:T4)
                n1432 = Unbundle(w2703) -> ("STATUS"=w2704:string)  [unwired: 2 out]
                n1433 = Equal?(x=w2704, y="RUN") -> (x = y?=w2700:bool)
                n1434 = And(x=w2700, y=w2701) -> (x .and. y?=w2699:bool)
                n1435 = case shown="True" w2699 {
                  tunnel: w2703 -> [_ w2707]
                  tunnel: w2697 -> [_ w2710]
                  frame False {
                  }
                  frame True {
                    n1436 = local read "SET LAB03-2"() -> (w2709:T5)
                    n1437 = local read "TDMS LAB03-2"() -> (w2706:refnum<k34>)
                    n1438 = Unbundle(w2707) -> ("CYCLE"=w2711:dbl)  [unwired: 2 out]
                    n1439 = Unbundle(w2709) -> ("T-RISE mins"=w2708:dbl)  [unwired: 4 out]
                    n1440 = Greater Or Equal?(x=w2711, y=w2710) -> (x >= y?=w2712:bool)
                    n1441 = case shown="True" w2712 {
                      tunnel: w2708 -> [w2715 _]
                      tunnel: w2707 -> [w2714 _]
                      tunnel: w2706 -> [w2713 _]
                      frame True {
                        n1442 = stacked-sequence {
                          tunnel: w2715 -> [w2718 _]
                          tunnel: w2714 -> [_ w2723]
                          tunnel: w2713 -> [w2716 _]
                          frame #0 {
                            n1443 = Build Array("T-RISE") -> (w2720:string[])
                            n1444 = Build Array(w2718) -> (w2719:dbl[])
                            n1445 = TDMS Write(0:w2716, 5:"TEST PASS", 7:w2720, 9:w2719) -> (15:w2722:errorcluster)  [unwired: 2 in, 3 out]
                            n1446 = local write "data file error"(w2722) -> ()
                          }
                          frame #1 {
                            n1447 = Bundle(cluster=w2723, "STATUS"="T-RISE PASS") -> (w2725:T4)  [unwired: 2 in]
                            n1448 = local write "RESULT LAB03-2"(TRUE) -> ()
                            n1449 = local write "DISP LAB03-2"(w2725) -> ()
                          }
                        }
                      }
                      frame False {
                      }
                    }
                  }
                }
              }
              frame #6 {
                # "LAB04-1"
                n1450 = Equal?(x=w2728, y=2) -> (x = y?=w2731:bool)
                n1451 = local read "DISP LAB04-1"() -> (w2733:T4)
                n1452 = Unbundle(w2733) -> ("STATUS"=w2734:string)  [unwired: 2 out]
                n1453 = Equal?(x=w2734, y="RUN") -> (x = y?=w2730:bool)
                n1454 = And(x=w2730, y=w2731) -> (x .and. y?=w2729:bool)
                n1455 = case shown="True" w2729 {
                  tunnel: w2733 -> [_ w2737]
                  tunnel: w2727 -> [_ w2740]
                  frame False {
                  }
                  frame True {
                    n1456 = local read "SET LAB04-1"() -> (w2739:T5)
                    n1457 = local read "TDMS LAB04-1"() -> (w2736:refnum<k34>)
                    n1458 = Unbundle(w2737) -> ("CYCLE"=w2741:dbl)  [unwired: 2 out]
                    n1459 = Unbundle(w2739) -> ("T-RISE mins"=w2738:dbl)  [unwired: 4 out]
                    n1460 = Greater Or Equal?(x=w2741, y=w2740) -> (x >= y?=w2742:bool)
                    n1461 = case shown="True" w2742 {
                      tunnel: w2738 -> [w2745 _]
                      tunnel: w2737 -> [w2744 _]
                      tunnel: w2736 -> [w2743 _]
                      frame True {
                        n1462 = stacked-sequence {
                          tunnel: w2745 -> [w2748 _]
                          tunnel: w2744 -> [_ w2753]
                          tunnel: w2743 -> [w2746 _]
                          frame #0 {
                            n1463 = Build Array("T-RISE") -> (w2750:string[])
                            n1464 = Build Array(w2748) -> (w2749:dbl[])
                            n1465 = TDMS Write(0:w2746, 5:"TEST PASS", 7:w2750, 9:w2749) -> (15:w2752:errorcluster)  [unwired: 2 in, 3 out]
                            n1466 = local write "data file error"(w2752) -> ()
                          }
                          frame #1 {
                            n1467 = Bundle(cluster=w2753, "STATUS"="T-RISE PASS") -> (w2755:T4)  [unwired: 2 in]
                            n1468 = local write "RESULT LAB04-1"(TRUE) -> ()
